vi "XNET Wait (Ethernet Synced).vi"(0 "session in":refnum<k21>, 7 "timeout (10)":dbl=10.0 format="%0.2f", 11 "error in (no error)":errorcluster) -> (4 "session out":refnum<k21>, 15 "error out":errorcluster)   [LabVIEW 2018]
doc: "Waits for the Ethernet interface to synchronize time on the network."
uses:
  nixlvapi.dll
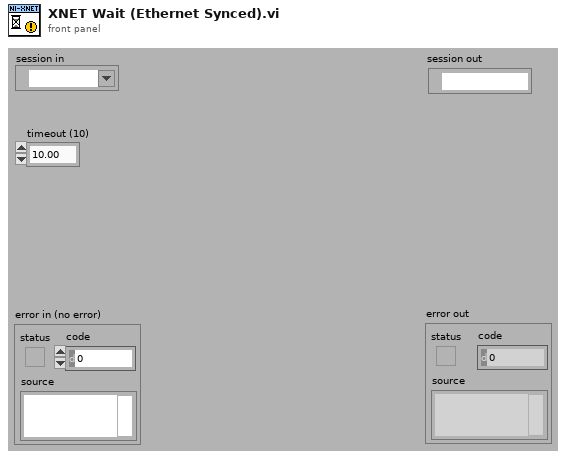
[diagram p1: front panel]
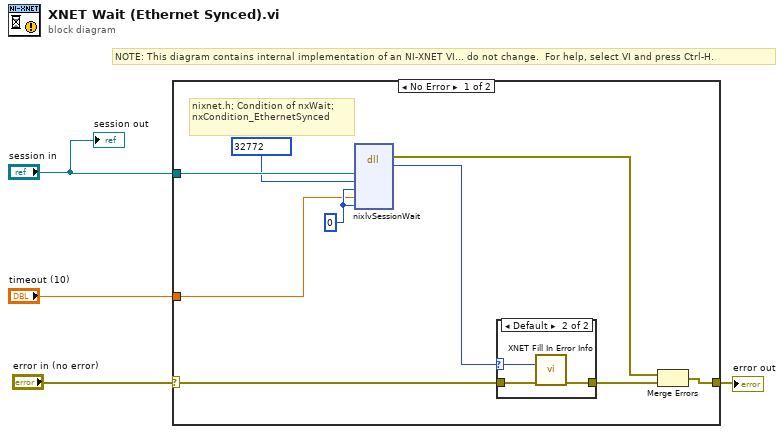
[diagram p0: block diagram]
diagram:
  # "NOTE: This diagram contains internal implementation of an NI-XNET VI... do not change.  For help, select VI and press Ctrl-H."
  n1 = case shown="No Error" "error in (no error)" {
    selector: "error in (no error)" -> [w13 w18]
    tunnel: "session in" -> [w11 _]
    tunnel: [w6 w18] -> w4
    tunnel: "timeout (10)" -> [w7 _]
    frame No Error {
      w8 = u32 0 ("ParamOut")
      # "nixnet.h; Condition of nxWait; nxCondition_EthernetSynced"
      # "NOTE: This diagram contains internal implementation of an NI-XNET VI... do not change.  For help, select VI and press Ctrl-H."
      n2 = dll-call lib="nixlvapi.*" fn="nixlvSessionWait" ("nilvxaiu.dll:lvxenSessionClear")("Reference"=w11, "Condition"=u32 32772 ("ParamOut"), "ParamIn"=w8, "Timeout"=w7, "ParamOut"=w8) -> (error out=w5:errorcluster, "return type"=w10:i32)  [unwired: 6 in, 3 out]
      n3 = case shown="Default" w10 {
        selector: w10 -> [_ w15]
        tunnel: w13 -> [w14 w16]
        tunnel: [w14 w17] -> w12
        frame 0 {
        }
        frame Default {
          n4 = call "XNET Fill In Error Info.vi"("status code"=w15, "error in"=w16) -> ("error out"=w17:errorcluster)  [unwired: 13 out]
        }
      }
      n5 = Merge Errors(w5, w12) -> (w6:errorcluster)
    }
    frame Error {
    }
  }
  "error out" <- w4
  "session out" <- "session in"
